vi "Data_structures_001.vi"() -> ()   [LabVIEW 2019]
uses:
  <vilib>/Math Plots/3D Math Plots/3D Surface/3D Surface XCtrl/3D Surface.xctl
  <vilib>/Math Plots/3D Math Plots/3D Surface/3D Surface Datatype/Public/Plot Helper (Matrix).vi
  <vilib>/Math Plots/3D Math Plots/3D Surface/3D Surface Datatype/3D Surface Datatype.lvclass
panel:
  in  "length 1":i32=3
  in  "index 1":i32=1
  in  "length 0":i32=1
  in  "index 0":i32
  out "Subarray of Double Control Array 2D":dbl[][](array[numeric])
  out "size 2":i32[](array[numeric])
  in  "Double Control Array 2D":dbl[][](array[numeric])=[[0.0, 1.55, 0.0, 0.0, 0.0, 0.0, 10.0], [0.0, 0.0, 0.0, 0.0, 0.0, 0.0, 0.0], [0.0, 0.0, 0.0, 7.0, 0.0, 0.0, 0.0]]
  out "3D Surface":refnum<class "3D Plot Datatype.lvclass">[](xcontrol)
  out "size 3":i32[](array[numeric])
  out "size 1":i32
  in  "String Control Array 2D":string[][](array[string])=[["Graphical", "Programming", "Course", "", "for", "PhD "], ["", "", "", "", "", ""], ["", "", "", "", "", ""], ["", "", "", "", "early", ""]]
  in  "Double Control Array 3D":dbl[][][](array[numeric])=[[[0.0, 1.55, 0.0, 0.0, 0.0, 0.0, 10.0], [0.0, 0.0, 0.0, 0.0, 0.0, 0.0, 0.0], [0.0, 0.0, 0.0, 7.0, 0.0, 0.0, 0.0]]]
  out "String Indicator Array":string[](array[string])
  out "Boolean Indicator Array":bool[](array[boolean])
  out "Int32 Indicator Array 2":i32[](array[numeric])
  out "Double Indicator Array":dbl[][](array[numeric])
  in  "Boolean Control Array":bool[](array[boolean])
  in  "Int32 Control Array":i32[](array[numeric])
  in  "String Control Array":string[](array[string])=["Graphical", "Programming", "Course", "", "for", "PhD "]
  in  "Double Control Array":dbl[](array[numeric])=[0.0, 1.55, 0.0, 0.0, 0.0, 0.0, 10.0]
  # "height"
  # "rows"
  # "columns"
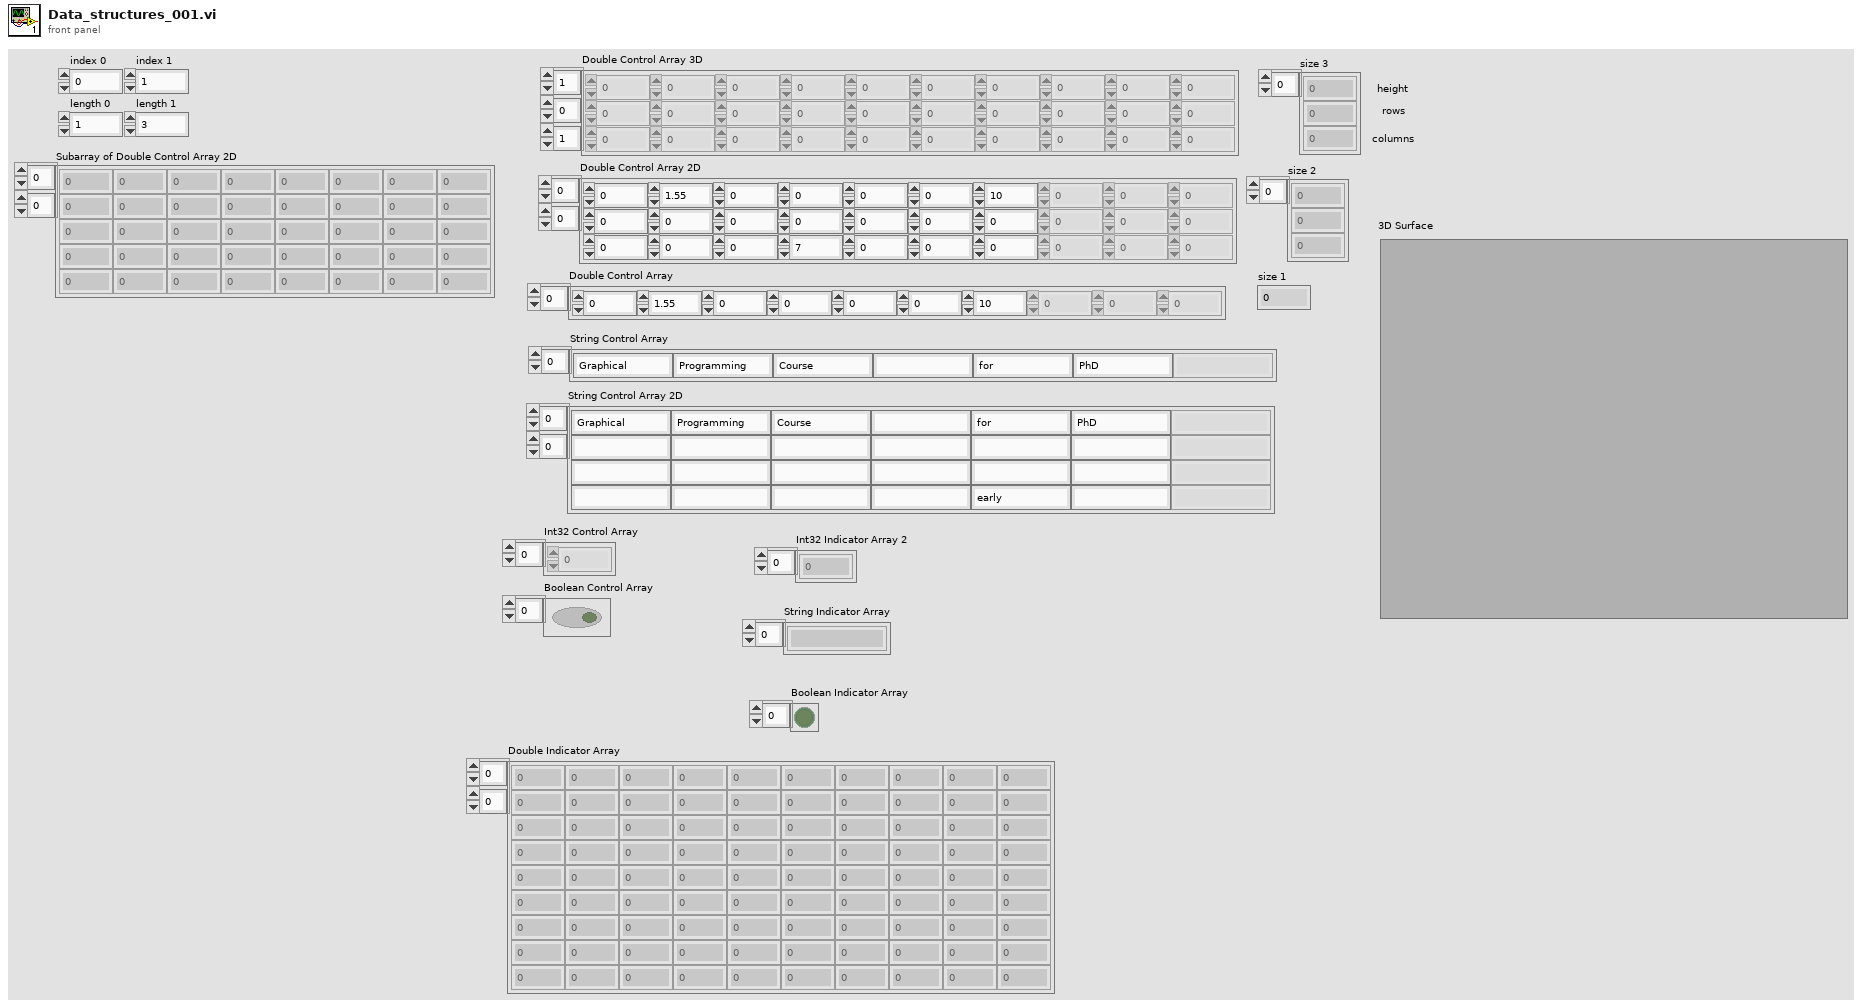
[diagram p1: front panel]
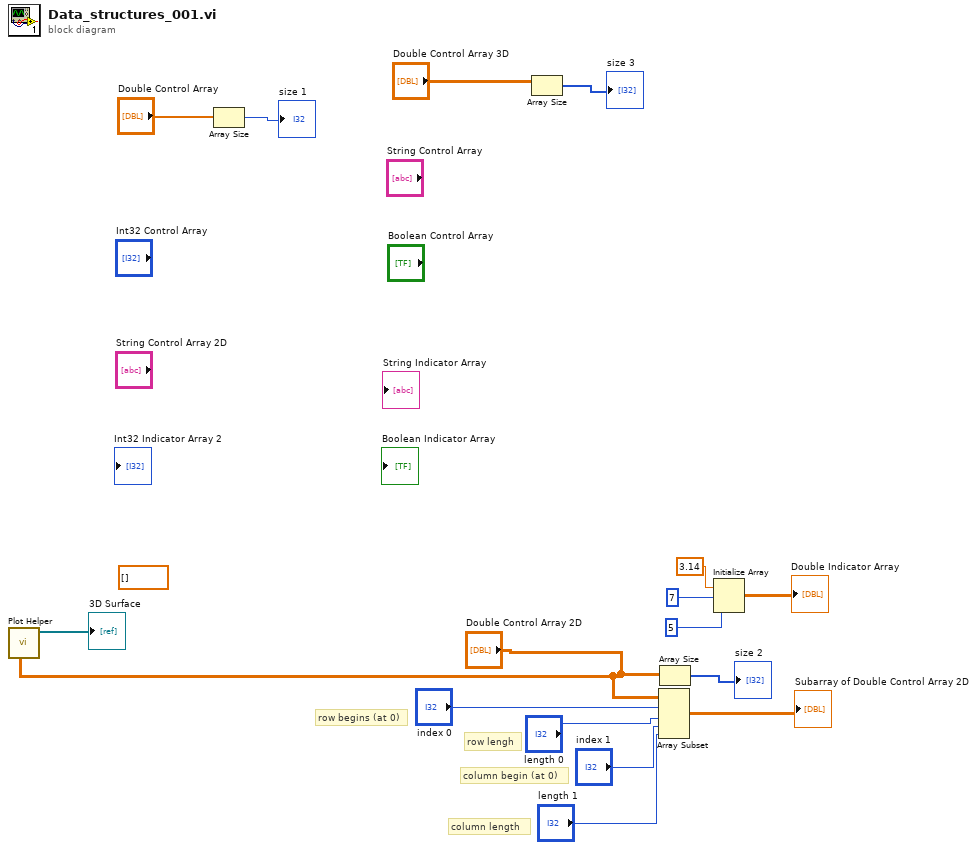
[diagram p0: block diagram]
diagram:
  (unwired) dbl[] []
  # "column length"
  # "column begin (at 0)"
  # "row lengh"
  # "row begins (at 0)"
  n1 = call-poly <vilib>:"Plot Helper.vi"("z matrix"="Double Control Array 2D") -> ("3D Plot lvclass Array out"=→"3D Surface":refnum<class "3D Plot Datatype.lvclass">[])  [unwired: 5 in, 5 out]
  n2 = Array Size(array="Double Control Array") -> (size(s)=→"size 1":i32)
  n3 = Array Size(array="Double Control Array 3D") -> (size(s)=→"size 3":i32[])
  n4 = Array Subset(array="Double Control Array 2D", index (row)="index 0", length (row)="length 0", index (col)="index 1", length (col)="length 1") -> (→"Subarray of Double Control Array 2D":dbl[][])
  n5 = Array Size(array="Double Control Array 2D") -> (size(s)=→"size 2":i32[])
  n6 = Initialize Array(3.14 ("element"), 7 ("dimension size"), 5 ("dimension size")) -> (→"Double Indicator Array":dbl[][])
